vi "SetTool.vi"(8 "error in":errorcluster, 11 "percent":dbl) -> (0 "error out":errorcluster)   [LabVIEW 2013]
panel:
  # "Note: This won't work\nBaxter needs a delay for \ngripper to move"
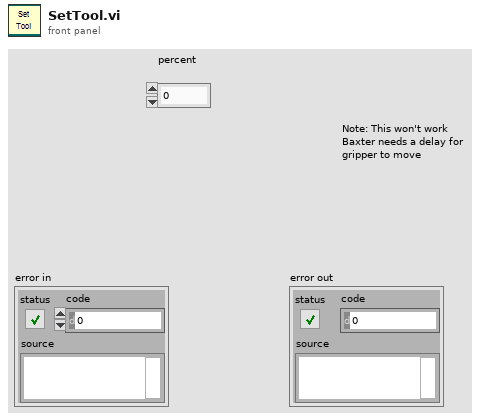
[diagram p1: front panel]
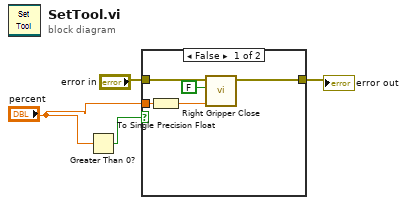
[diagram p0: block diagram]
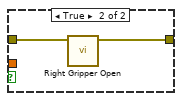
[diagram p2: hidden frame]
diagram:
  n1 = Greater Than 0?(x="percent") -> (x > 0?=w1:bool)
  n2 = case shown="False" w1 {
    tunnel: "error in" -> [w9 w10]
    tunnel: [w8 w11] -> w3
    tunnel: "percent" -> [w6 _]
    frame False {
      n3 = To Single Precision Float(number=w6) -> (single precision float=w5:sgl)
      n4 = call "Right Gripper Close.vi"("Target Position"=w5, "Pause on Miss?"=FALSE, "error in"=w9) -> ("error out"=w8:errorcluster)  [unwired: 7 in, 1 out]
    }
    frame True {
      n5 = call "Right Gripper Open.vi"("error in"=w10) -> ("error out"=w11:errorcluster)  [unwired: 10 in]
    }
  }
  "error out" <- w3
